vi "TurnAngle.vi"(2 "WristMode":bool=TRUE, 3 "LiftMode":bool=TRUE, 5 "Intake":dbl format="%#_13g", 6 "Lift":dbl format="%#_13g", 7 "Wrist":dbl format="%#_13g", 8 "Time":dbl=5.0 format="%#_13g", 9 "AngleSetpoint":dbl format="%#_13g", 10 "MaxSpeed":dbl) -> ()   [LabVIEW 2017]
uses:
  Phoenix-LabVIEW/Motor Controller/Controls/CTRE_Phoenix_MotorControl_ControlMode.ctl
panel:
  in  "PID_NAVX":T1={"proportional gain (Kc)"=0.03, "integral time (Ti, min)"=0.0, "derivative time (Td, min)"=0.0}
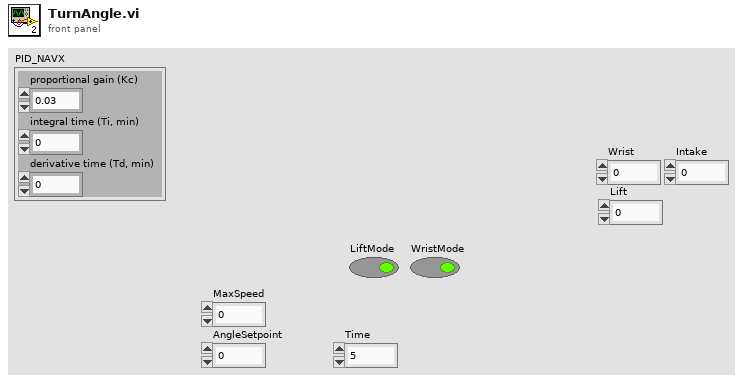
[diagram p1: front panel]
types:
  T1 = cluster{"proportional gain (Kc)":dbl, "integral time (Ti, min)":dbl, "derivative time (Td, min)":dbl}
  T2 = typedef "CTRE_Phoenix_MotorControl_ControlMode.ctl" = u16
  T3 = typedef "WPI_MotorControlDeviceRef.ctl" = cluster{"DeviceStatus":errorcluster, "Type":T4, "PWM":cluster{"PWM Channel":T5, "DeadBand":T6}, "CAN":cluster{"Device Number":u8, "SetOutput VI Ref":variant, "GetOutput VI Ref":variant, "Enable VI Ref":variant, "Disable VI Ref":variant, "Data":variant}, "Invert":bool, "DIO PWM":cluster{"PWM \"Enable\" Channel":T5, "DIOChannel":T7, "PWM Rate":dbl}}
  T4 = typedef "WPI_MotorControlType.ctl" = enum16{"PWM", "CAN", "DIO PWM"}
  T5 = typedef "FPGA_DIOPWMChannel.ctl" = enum8{"PWM 0", "PWM 1", "PWM 2", "PWM 3", "PWM 4", "PWM 5", "PWM 6", "PWM 7", "PWM 8", "PWM 9", "PWM MXP 0", "PWM MXP 1", "PWM MXP 2", "PWM MXP 3", "PWM MXP 4", "PWM MXP 5", "PWM MXP 6", "PWM MXP 7", "PWM MXP 8", "PWM MXP 9", "Invalid"}
  T6 = typedef "WPI_PWMDeadband.ctl" = cluster{"Name":string, "maxPositivePwm":i32, "minPositivePwm":i32, "centerPwm":i32, "maxNegativePwm":i32, "minNegativePwm":i32, "angularRange":u16}
  T7 = typedef "FPGA_DIOChannel.ctl" = enum8{"DIO 0", "DIO 1", "DIO 2", "DIO 3", "DIO 4", "DIO 5", "DIO 6", "DIO 7", "DIO 8", "DIO 9", "DIO MXP 0", "DIO MXP 1", "DIO MXP 2", "DIO MXP 3", "DIO MXP 4", "DIO MXP 5", "DIO MXP 6", "DIO MXP 7", "DIO MXP 8", "DIO MXP 9", "DIO MXP 10", "DIO MXP 11", "DIO MXP 12", "DIO MXP 13", "DIO MXP 14", "DIO MXP 15", "SPI Port CS1", "SPI Port CS2", "SPI Port CS3", "SPI Port MISO", "SPI Port MOSI", "Invalid"}
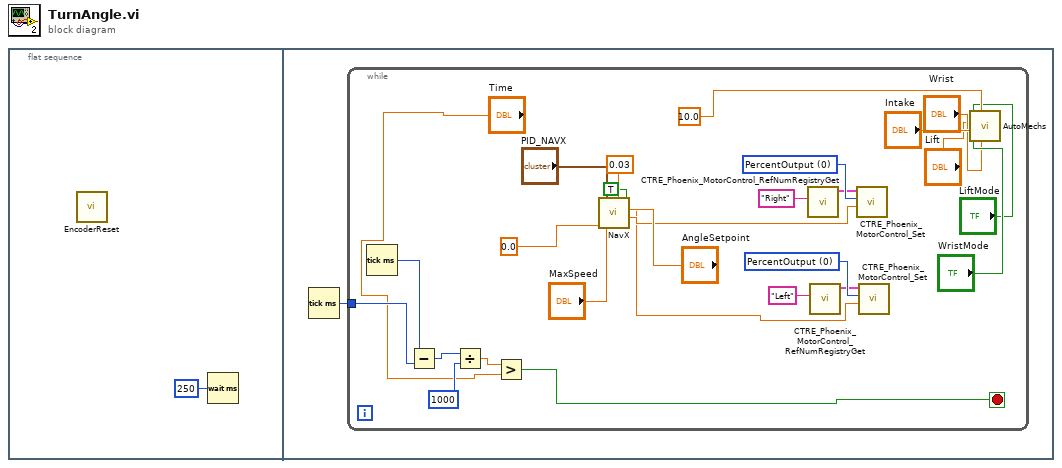
[diagram p0: block diagram]
diagram:
  n1 = flat-sequence {
    frame #0 {
      n2 = call "EncoderReset.vi"() -> ()  [unwired: 12 in]
      n3 = Wait (ms)(milliseconds to wait=u32 250) -> ()  [unwired: 1 out]
    }
    frame #1 {
      n4 = Tick Count (ms)() -> (millisecond timer value=w2:u32)
      n5 = while {
        tunnel: w2 -> [w9]
        stop <- w7 stop-if-true
        w21 = T2 0 items=["PercentOutput"=0, "Position"=1, "Velocity"=2, "Current"=3, "Follower"=5, "MotionProfile"=6, "MotionMagic"=7, "MotionMagicArc"=8, "MotionProfileArc"=10, "Disabled"=15] ("Control Mode")
        w24 = T2 0 items=["PercentOutput"=0, "Position"=1, "Velocity"=2, "Current"=3, "Follower"=5, "MotionProfile"=6, "MotionMagic"=7, "MotionMagicArc"=8, "MotionProfileArc"=10, "Disabled"=15] ("Control Mode")
        n6 = Tick Count (ms)() -> (millisecond timer value=w13:u32)
        n7 = Subtract(x=w13, y=w9) -> (x-y=w12:u32)
        n8 = Divide(x=w12, y=u32 1000) -> (x/y=w10:dbl)
        n9 = Greater?(x=w10, y="Time") -> (0:w7:bool)
        n10 = call "NavX.vi"("PID gains"="PID_NAVX", "AngleSetpoint"="AngleSetpoint", "MaxSpeed"="MaxSpeed", "NavxSpeed"=0.0, "NavX_P"=0.03, "PID?"=TRUE) -> ("LeftNavx"=w16:dbl, "RightNavx"=w18:dbl)  [unwired: 1 out]
        n11 = call "CTRE_Phoenix_MotorControl_RefNumRegistryGet.vi"("refnum name"="Right") -> ("PhoenixMotorControlDevRef"=w20:T3)  [unwired: 9 in, 1 out]
        n12 = call "CTRE_Phoenix_MotorControl_RefNumRegistryGet.vi"("refnum name"="Left") -> ("PhoenixMotorControlDevRef"=w23:T3)  [unwired: 9 in, 1 out]
        n13 = call "CTRE_Phoenix_MotorControl_Set.vi"("Output"=w18, "Control Mode"=w21, "PhoenixMotorControlDevRef"=w20) -> ()  [unwired: 7 in, 2 out]
        n14 = call "CTRE_Phoenix_MotorControl_Set.vi"("Output"=w16, "Control Mode"=w24, "PhoenixMotorControlDevRef"=w23) -> ()  [unwired: 7 in, 2 out]
        n15 = call "AutoMechs.vi"("Wrist"="Wrist", "Time"=10.0, "WristMode"="WristMode", "Intake"="Intake", "Lift"="Lift", "LiftMode"="LiftMode") -> ()  [unwired: 6 in]
      }
    }
  }
